vi "send_freq.vi"(3 "error in (no error)":errorcluster, 4 "elemszam":u8, 5 "signal freq":u32, 6 "VISA Refnum in":refnum<visa-resource-name>) -> (0 "error out":errorcluster, 1 "VISA Refnum out":refnum<visa-resource-name>, 2 "tmr 2 rld value":u16)   [LabVIEW 2014]
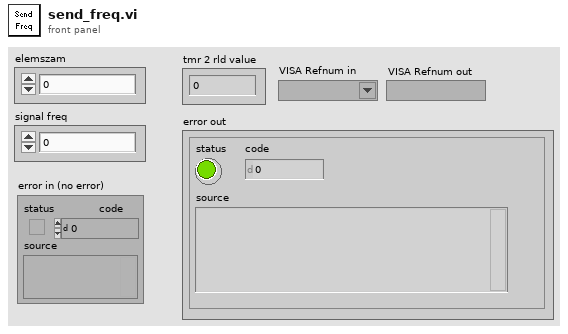
[diagram p1: front panel]
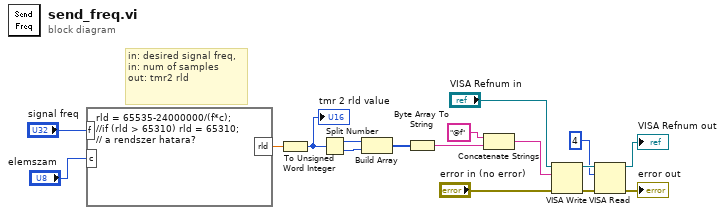
[diagram p0: block diagram]
diagram:
  # "in: desired signal freq, \nin: num of samples\nout: tmr2 rld"
  n1 = formula code="rld = 65535-24000000/(f*c);\n//if (rld > 65310) rld = 65310;\n// a rendszer hatara?"("f"="signal freq", "c"="elemszam") -> ("rld"=w3:dbl)
  n2 = To Unsigned Word Integer(number=w3) -> (unsigned 16bit integer=w2:u16)
  "tmr 2 rld value" <- w2
  n3 = Split Number(x=w2) -> (hi(x)=w14:u8, lo(x)=w15:u8)
  n4 = Build Array(w14, w15) -> (w16:u8[])
  n5 = Byte Array To String(unsigned byte array=w16) -> (string=w17:string)
  n6 = Concatenate Strings("@f" ("write buffer"), w17) -> (w8:string)
  n7 = VISA Write(VISA resource name="VISA Refnum in", write buffer=w8, error in (no error)="error in (no error)") -> (VISA resource name out=w10:refnum<visa-resource-name>, error out=w11:errorcluster)  [unwired: 1 out]
  n8 = VISA Read(VISA resource name=w10, byte count=u32 4, error in (no error)=w11) -> (VISA resource name out=→"VISA Refnum out":refnum<visa-resource-name>, error out=→"error out":errorcluster)  [unwired: 2 out]
